vi "Read Acquire Pulse Ref.vi"(8 "error in (no error)":errorcluster, 11 "Measure Pulse in":refnum<class "Measure Pulse.lvclass">) -> (0 "error out":errorcluster, 2 "Acquire Pulse Ref":refnum<vi>, 3 "Measure Pulse out":refnum<class "Measure Pulse.lvclass">)   [LabVIEW 2015, in "Measure Pulse.lvclass"]
uses:
  Measure Pulse.lvclass
  Queued Listbox/Queued Listbox.xctl
  Measure Pulse.lvclass/Measure Pulse.ctl
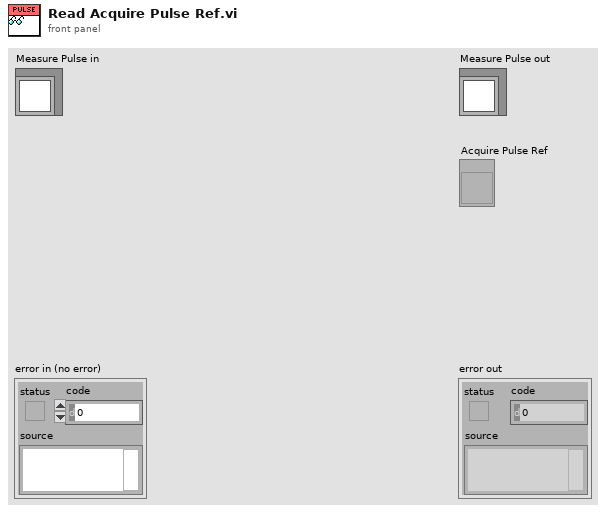
[diagram p1: front panel]
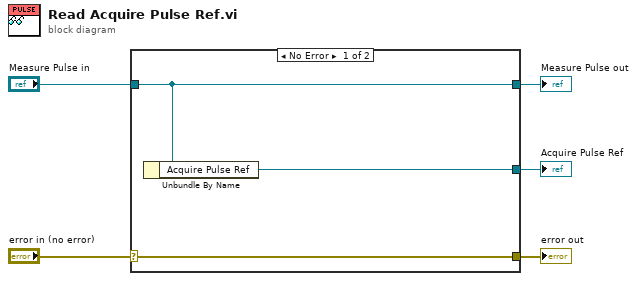
[diagram p0: block diagram]
diagram:
  n1 = case shown="No Error" "error in (no error)" {
    selector: "error in (no error)" -> [w8 w9]
    tunnel: [w8 w9] -> w4
    tunnel: [w7 w10] -> w2
    tunnel: "Measure Pulse in" -> [w7 w10]
    tunnel: [w6 _] -> w1
    frame No Error {
      n2 = Unbundle By Name(w7) -> ("Acquire Pulse Ref"=w6:refnum<vi>)
    }
    frame Error {
    }
  }
  "error out" <- w4
  "Measure Pulse out" <- w2
  "Acquire Pulse Ref" <- w1
